vi "Set Message Queue.vi"(8 "error in (no error)":errorcluster, 10 "Message Queue":refnum<queue>, 11 "Communication in":refnum<class "Message Transport.lvclass">) -> (0 "error out":errorcluster, 3 "Communication out":refnum<class "Message Transport.lvclass">)   [LabVIEW 2018, in "Message Transport.lvclass"]
uses:
  Message Transport_class/Message Transport.lvclass
  Message_class/Message.lvclass
  Message Transport_class/Message Transport.lvclass/Message Transport.ctl
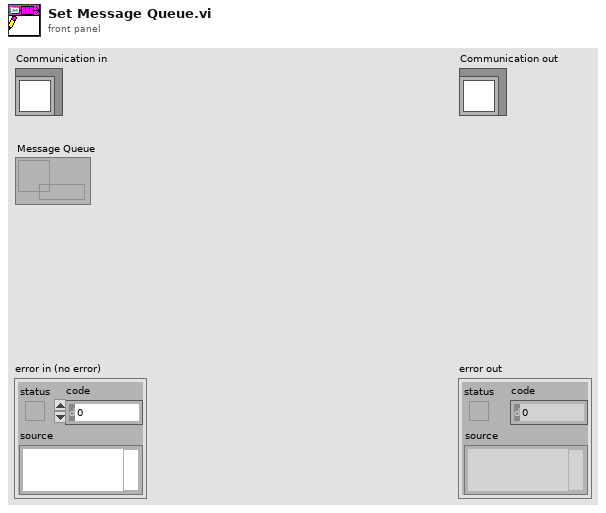
[diagram p1: front panel]
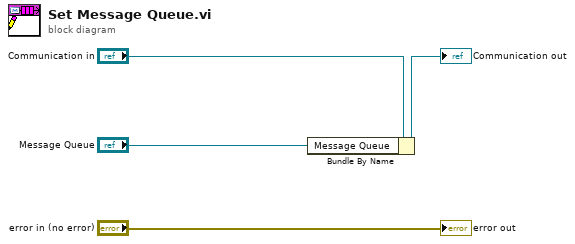
[diagram p0: block diagram]
diagram:
  n1 = Bundle By Name(cluster="Communication in", "Message Queue"="Message Queue") -> (→"Communication out":refnum<class "Message Transport.lvclass">)
  "error out" <- "error in (no error)"
